vi "T257P_Set_Temperature.vi"(0 "T257P Port IN":refnum<visa-resource-name>, 1 "Set Temperature (C)":dbl=20.0 format="%.2g", 5 "error in (no error)":errorcluster) -> (7 "Sent buffer 1":string, 11 "Read buffer 1":string, 14 "T257P Port OUT":refnum<visa-resource-name>, 15 "Set Temperature (C)":dbl format="%.2f", 16 "CheckSum 1":string, 19 "error out":errorcluster)   [LabVIEW 2020]
doc: "ThermoTek T257P Labview Driver Library. © G.Shtengel. gleb.shtengel@gmail.com"
panel:
  out "Loop Counter 1":i32
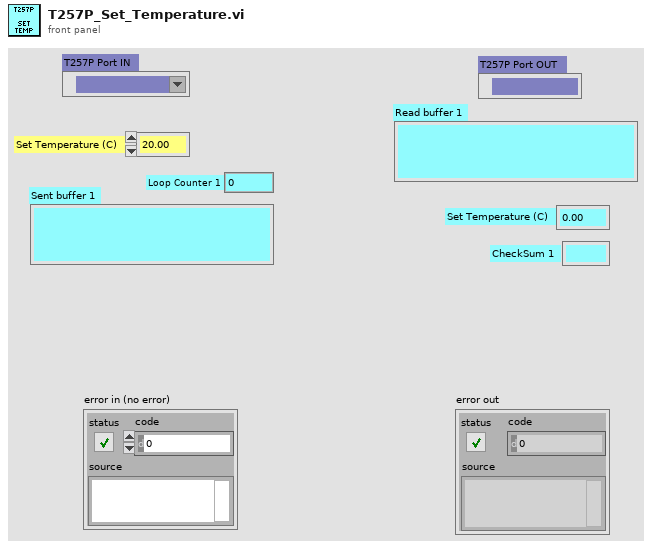
[diagram p1: front panel]
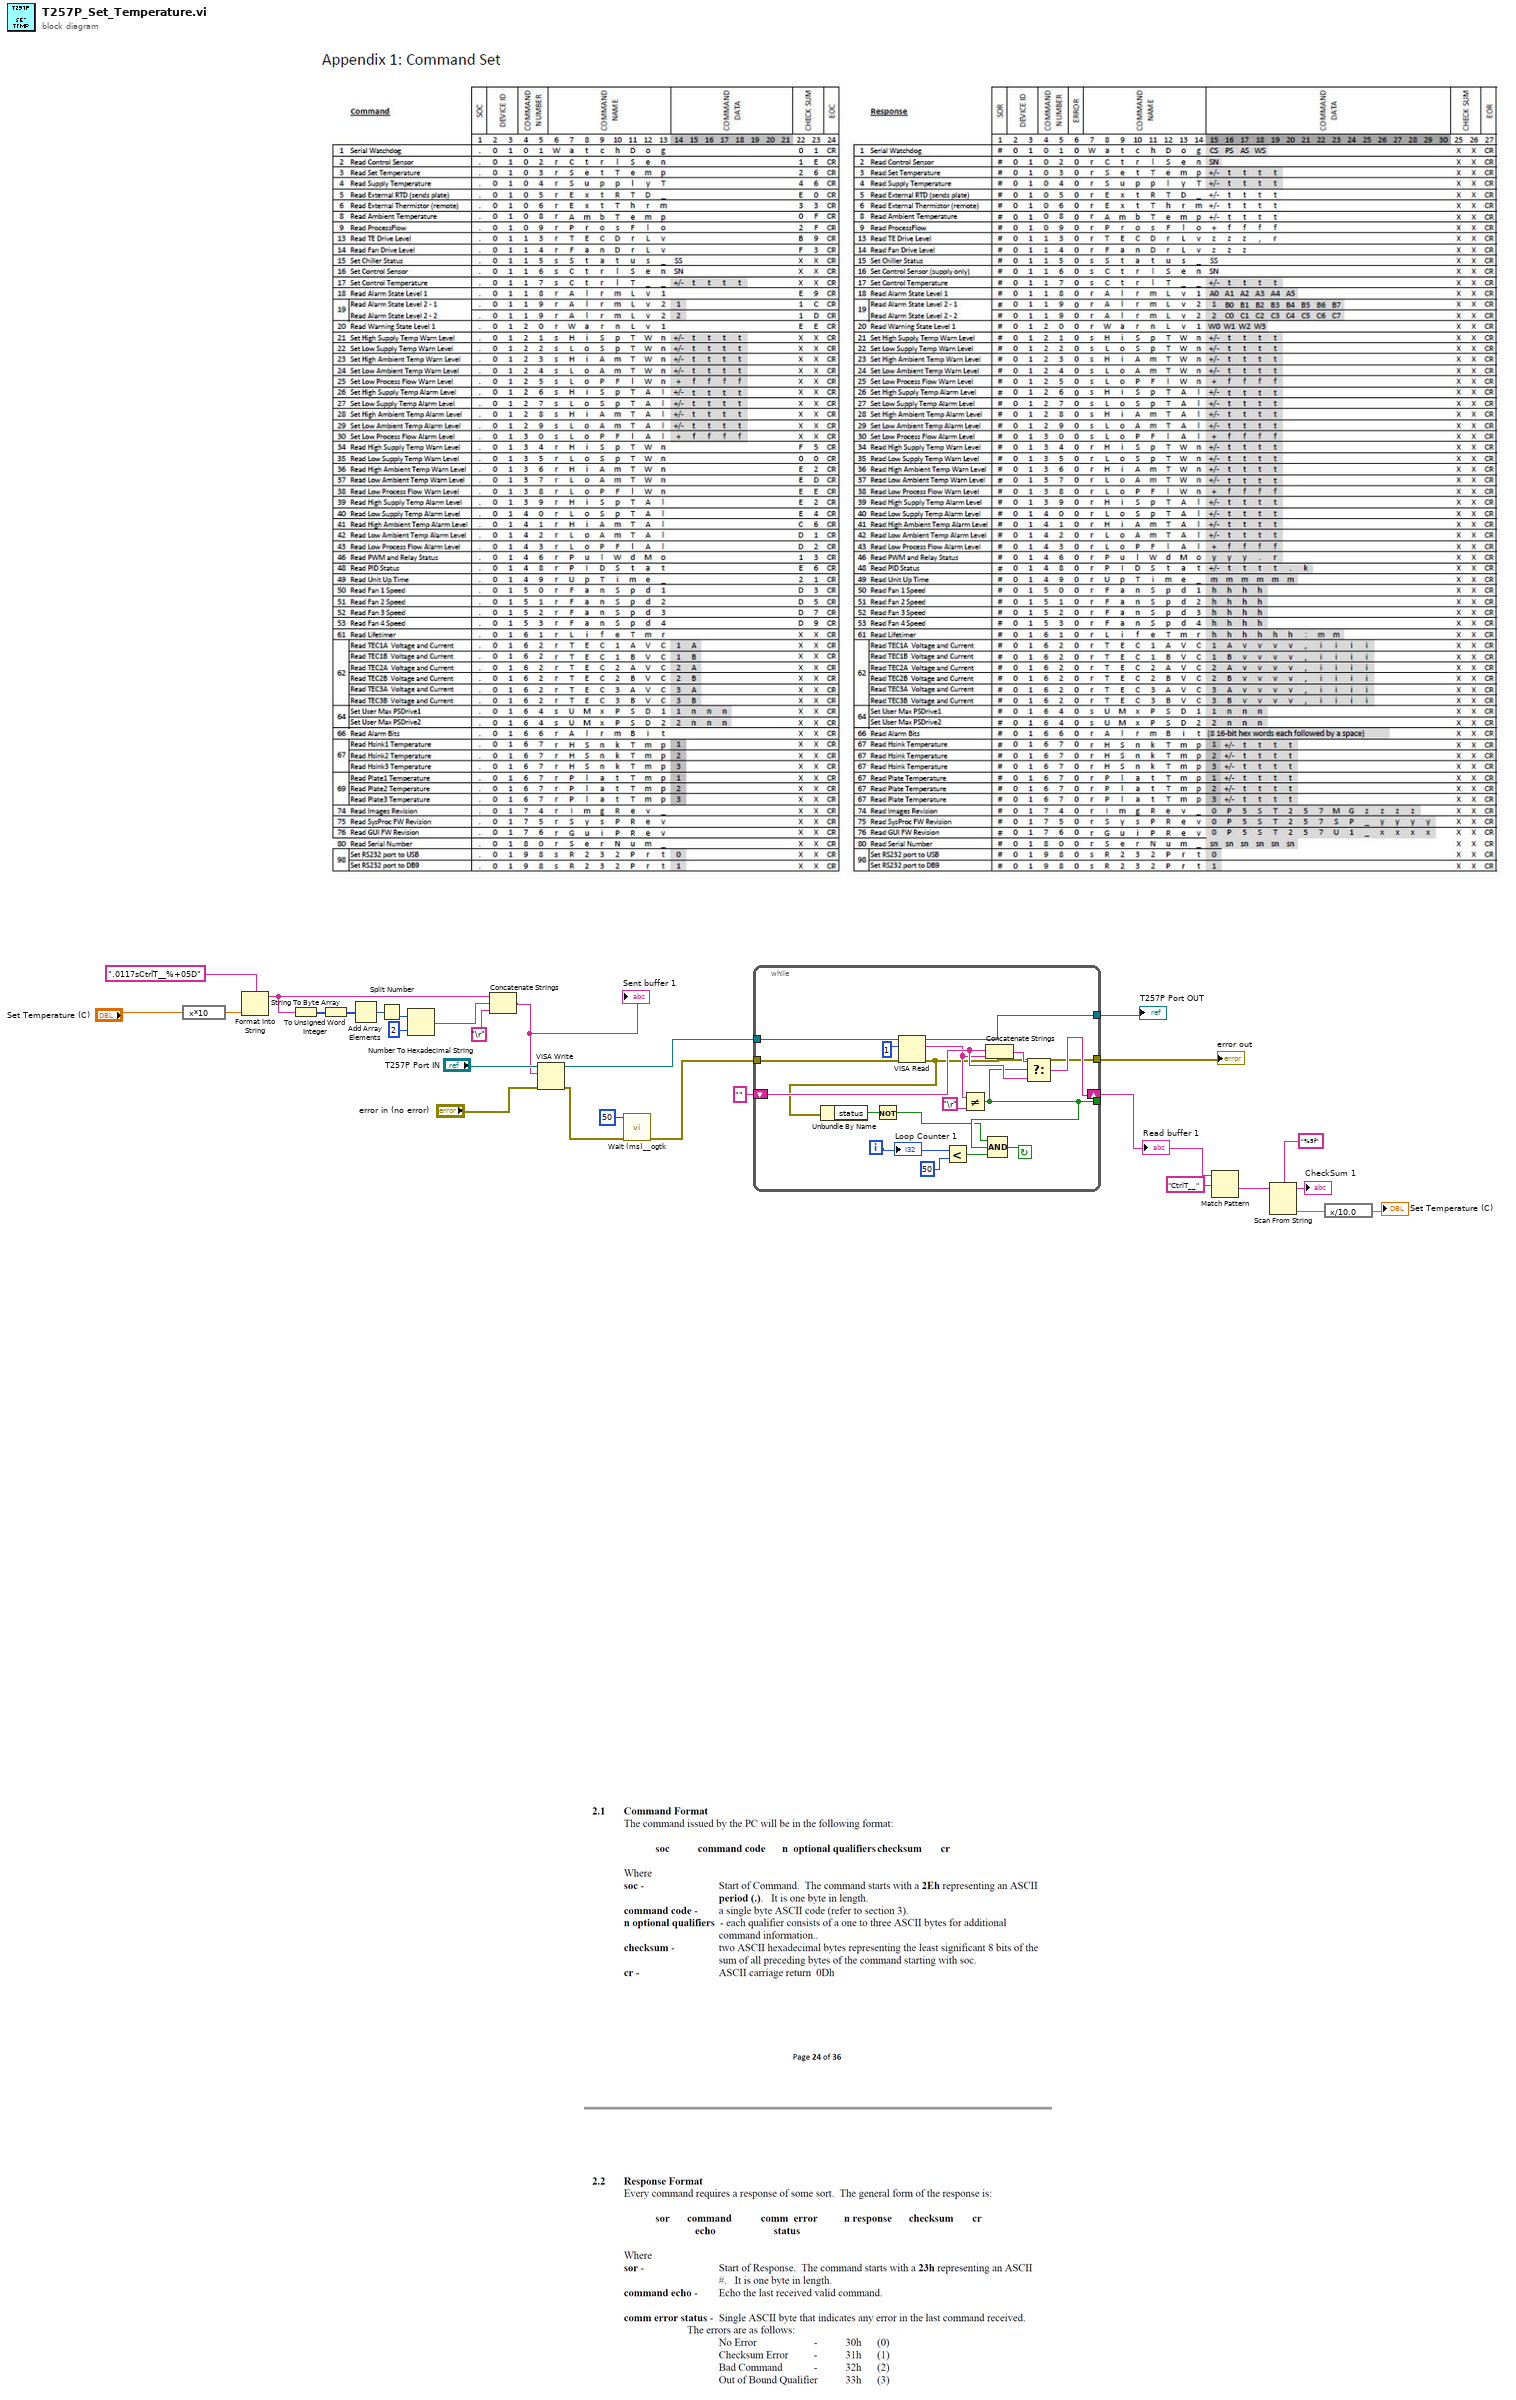
[diagram p0: block diagram]
diagram:
  n1 = expression code="x*10"("Set Temperature (C)") -> (w5:dbl)
  n2 = Format Into String(format string=".0117sCtrlT__%+05D" ("Sent buffer 2"), w5) -> (resulting string=w8:string)  [unwired: 2 in, 1 out]
  n3 = String To Byte Array(string=w8) -> (unsigned byte array=w12:u8[])
  n4 = To Unsigned Word Integer(number=w12) -> (unsigned 16bit integer=w11:u16[])
  n5 = Add Array Elements(numeric array=w11) -> (sum=w10:u16)
  n6 = Split Number(x=w10) -> (lo(x)=w9:u8)  [unwired: 1 out]
  n7 = Number To Hexadecimal String(1:i16 2 ("width (-)"), 2:w9) -> (0:w7:string)
  n8 = Concatenate Strings(w8, w7, "\r") -> (w4:string)
  "Sent buffer 1" <- w4
  n9 = VISA Write(VISA resource name="T257P Port IN", write buffer=w4, error in (no error)="error in (no error)") -> (VISA resource name out=w24:refnum<visa-resource-name>, error out=w25:errorcluster)  [unwired: 1 out]
  n10 = call <userlib>:"Wait (ms)__ogtk.vi"("error in (no error)"=w25, "milliseconds to wait"=u32 50) -> ("error out"=w23:errorcluster)  [unwired: 8 in, 1 out]
  n11 = while {
    shift-left: "" -> [w42]
    shift-right: [w41] -> w18
    tunnel: [w39] -> _
    tunnel: [w31] -> w13
    tunnel: [w40] -> w14
    tunnel: w24 -> [w37]
    tunnel: w23 -> [w36]
    i -> [w38]
    stop <- w43 continue-if-true
    n12 = VISA Read(VISA resource name=w37, byte count=u32 1 ("byte count (0)"), error in (no error)=w36) -> (VISA resource name out=w40:refnum<visa-resource-name>, read buffer=w34:string, error out=w31:errorcluster)  [unwired: 1 out]
    n13 = Unbundle By Name(w31) -> ("status"=w30:bool)
    n14 = Not(x=w30) -> (.not. x?=w29:bool)
    n15 = Less?(x=w38, y=50) -> (x < y?=w44:bool)
    n16 = Not Equal?(x=w34, y="\r") -> (x != y?=w39:bool)
    n17 = Concatenate Strings(w42, w34) -> (w32:string)
    n18 = Compound Arithmetic op=AND(w29, w39, w44) -> (w43:bool)
    n19 = Select(t=w32, s=w39, f=w42) -> (s? t:f=w41:string)
    "Loop Counter 1" <- w38
  }
  "error out" <- w13
  "Read buffer 1" <- w18
  "T257P Port OUT" <- w14
  n20 = Match Pattern(string=w18, regular expression="CtrlT__") -> (after substring=w19:string)  [unwired: 1 in, 3 out]
  n21 = Scan From String(format string="%5f", input string=w19) -> (remaining string=→"CheckSum 1":string, output 1=w17:dbl)  [unwired: 3 in, 2 out]
  n22 = expression code="x/10.0"(w17) -> (→"Set Temperature (C)":dbl)
